vi "ShooterAngleControl.vi"(3 "error in (no error)":errorcluster, 4 "Zero":bool, 5 "Rotations":dbl) -> (0 "error out":errorcluster)   [LabVIEW 2012]
uses:
  <vilib>/Rock Robotics/WPI/CAN/Jaguar/SubVIs/WPI_CANJaguar_ControlMode.ctl
  <vilib>/Rock Robotics/WPI/CAN/Jaguar/SubVIs/WPI_CANJaguar_StatusSelect.ctl
  <vilib>/Rock Robotics/WPI/SafetyOutput/WPI_SafetyOutputConfigMenu.ctl
  <vilib>/Rock Robotics/WPI/CAN/Jaguar/SubVIs/WPI_CANJaguar_StatusChannelSelect.ctl
  Robot Global Data.vi
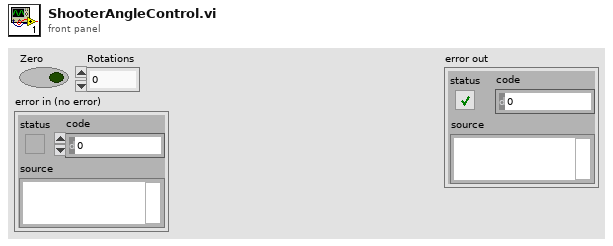
[diagram p1: front panel]
types:
  T1 = typedef "WPI_MotorControlDeviceRef.ctl" = cluster{"DeviceStatus":errorcluster, "Type":enum16{"PWM", "CAN"}, "PWM":cluster{"Digital Module":T2, "PWM Channel":T3, "DeadBand":T4}, "CAN":cluster{"Device Number":u8, "Control Mode":T5, "Semaphore":T6, "Max Vout":dbl}, "Invert":bool, "TransformRef":T7, "InvTransformRef":T7}
  T2 = typedef "FPGA_TypedefDigitalModule.ctl" = enum16{"Digital Module 1", "Digital Module 2"}
  T3 = typedef "FPGA_DIOPWMChannel.ctl" = enum8{"PWM 1", "PWM 2", "PWM 3", "PWM 4", "PWM 5", "PWM 6", "PWM 7", "PWM 8", "PWM 9", "PWM 10", "Invalid"}
  T4 = typedef "WPI_PWMDeadband.ctl" = cluster{"Name":string, "maxPositivePwm":i32, "minPositivePwm":i32, "centerPwm":i32, "maxNegativePwm":i32, "minNegativePwm":i32, "angularRange":u16}
  T5 = typedef "WPI_CANJaguar_ControlMode.ctl" = enum8{"Percent VBus", "Current", "Speed", "Position", "Voltage"}
  T6 = typedef "Semaphore RefNum" = refnum<k1>
  T7 = typedef "WPI_PWMTransform_ConPane.ctl" = refnum<vi>
  T8 = typedef "WPI_CANJaguar_StatusChannelSelect.ctl" = enum16{"Periodic Status Channel 1", "Periodic Status Channel 2", "Periodic Status Channel 3", "Periodic Status Channel 4", "On Demand Status"}
  T9 = typedef "WPI_SafetyOutputConfigMenu.ctl" = enum16{"Enable", "Disable"}
  T10 = typedef "WPI_CANJaguar_StatusSelect.ctl" = enum16{"Output Percent VBus", "Output Voltage", "Bus Voltage", "Current", "Temperature", "Position", "Speed", "Limit Switches", "Faults", "Fault Counters", "Power Cycle"}
  T11 = typedef "WPI_CANJaguar_Status.ctl" = cluster{"Output Percent VBus":dbl, "Output Voltage":dbl, "Bus Voltage":dbl, "Current":dbl, "Temperature":dbl, "Position":dbl, "Speed":dbl, "Limits":cluster{"Forward Limit":bool, "Reverse Limit":bool, "Forward Soft Limit":bool, "Reverse Soft Limit":bool, "Sticky Forward Limit":bool, "Sticky Reverse Limit":bool, "Sticky Forward Soft Limit":bool, "Sticky Reverse Soft Limit":bool}, "Faults":cluster{"Current Fault":bool, "Temperature Fault":bool, "Bus Voltage Fault":bool, "Gate Driver Fault":bool, "Comm Fault":bool}, "Fault Counters":cluster{"Current Faults":u8, "Temperature Faults":u8, "Bus Voltage Faults":u8, "Gate Driver Faults":u8, "Comm Faults":u8, "CAN Status":u8, "CAN RX Errors":u8, "CAN TX Errors":u8}, "Power Cycle":bool}
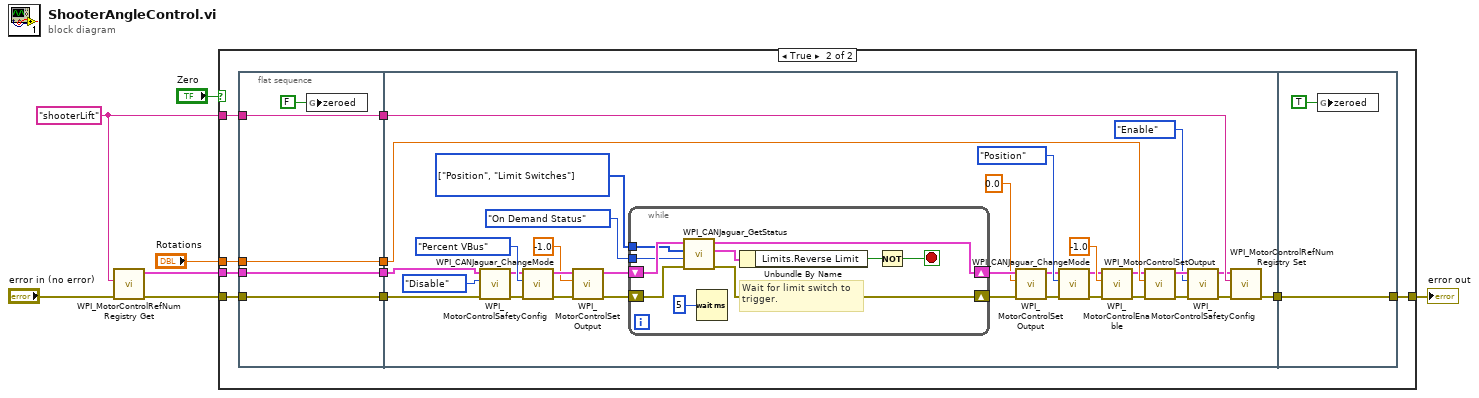
[diagram p0: block diagram]
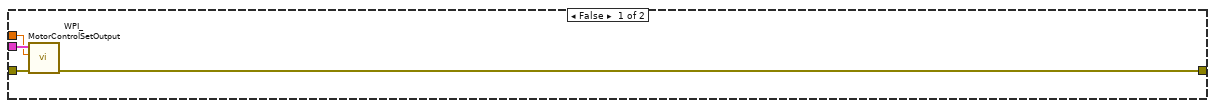
[diagram p2: hidden frame]
diagram:
  w1 = "shooterLift" ("refnum name")
  n1 = call <vilib>:"WPI_MotorControlRefNum Registry Get.vi"("error in (no error)"="error in (no error)", "refnum name"=w1) -> ("error out"=w7:errorcluster, "MotorControlDevRef"=w6:T1)  [unwired: 8 in]
  n2 = case shown="True" "Zero" {
    tunnel: w7 -> [w10 w17]
    tunnel: w6 -> [w11 w18]
    tunnel: [w9 w21] -> w3
    tunnel: "Rotations" -> [w8 w19]
    tunnel: w1 -> [_ w20]
    frame False {
      n3 = call <vilib>:"WPI_MotorControlSetOutput.vi"("error in (no error)"=w10, "Output"=w8, "MotorControlDevRef"=w11) -> ("error out"=w9:errorcluster)  [unwired: 6 in, 2 out]
    }
    frame True {
      n4 = flat-sequence {
        tunnel: w17 -> [w23]
        tunnel: w18 -> [w24]
        tunnel: w19 -> [w25]
        tunnel: w20 -> [w26]
        tunnel: [w26] -> w16
        tunnel: [w25] -> w15
        tunnel: [w24] -> w14
        tunnel: [w23] -> w13
        tunnel: w16 -> [w47]
        tunnel: w15 -> [w45]
        tunnel: w14 -> [w44]
        tunnel: w13 -> [w43]
        tunnel: [w48] -> w12
        tunnel: [w70] -> w21
        tunnel: w12 -> [w70]
        frame #0 {
          n5 = global write "Robot Global Data.vi" "zeroed"(FALSE ("zeroed")) -> ()
        }
        frame #1 {
          w52 = T10[] [enum."Position", enum."Limit Switches"] items=["Output Percent VBus", "Output Voltage", "Bus Voltage", "Current", "Temperature", "Position", "Speed", "Limit Switches", "Faults", "Fault Counters", "Power Cycle"] ("Status Select")
          n6 = call <vilib>:"WPI_MotorControlSafetyConfig.vi"("error in (no error)"=w43, "mode"=WPI_SafetyOutputConfigMenu."Disable", "MotorControlDevRef"=w44) -> ("error out"=w40:errorcluster, "MotorControlDevRef"=w41:T1)  [unwired: 7 in]
          n7 = call <vilib>:"WPI_CANJaguar_ChangeMode.vi"("error in (no error)"=w40, "Control Mode"=WPI_CANJaguar_ControlMode."Percent VBus", "CAN Jaguar Ref"=w41) -> ("error out"=w57:errorcluster, "CAN Jaguar Ref Out"=w56:T1)  [unwired: 7 in]
          n8 = call <vilib>:"WPI_MotorControlSetOutput.vi"("error in (no error)"=w57, "Output"=-1.0, "MotorControlDevRef"=w56) -> ("error out"=w54:errorcluster, "MotorControlDevRef"=w53:T1)  [unwired: 6 in, 1 out]
          n9 = while {
            tunnel: w52 -> [w65]
            shift-right: [w64] -> w49
            shift-left: w53 -> [w67]
            shift-right: [w63] -> w50
            shift-left: w54 -> [w68]
            tunnel: WPI_CANJaguar_StatusChannelSelect."On Demand Status" ("Status Channel Select") -> [w60]
            stop <- w59 stop-if-true
            # "Wait for limit switch to\ntrigger."
            n10 = call <vilib>:"WPI_CANJaguar_GetStatus.vi"("error in (no error)"=w68, "Status Channel Select"=w60, "Status Select"=w65, "CAN Jaguar Ref"=w67) -> ("error out"=w63:errorcluster, "Status"=w66:T11, "CAN Jaguar Ref Out"=w64:T1)  [unwired: 5 in]
            n11 = Wait (ms)(milliseconds to wait=u32 5) -> ()  [unwired: 1 out]
            n12 = Unbundle By Name(w66) -> ("Limits.Reverse Limit"=w61:bool)
            n13 = Not(x=w61) -> (.not. x?=w59:bool)
          }
          n14 = call <vilib>:"WPI_MotorControlSetOutput.vi"("error in (no error)"=w50, "Output"=0.0, "MotorControlDevRef"=w49) -> ("error out"=w29:errorcluster, "MotorControlDevRef"=w28:T1)  [unwired: 6 in, 1 out]
          n15 = call <vilib>:"WPI_CANJaguar_ChangeMode.vi"("error in (no error)"=w29, "Control Mode"=WPI_CANJaguar_ControlMode."Position", "CAN Jaguar Ref"=w28) -> ("error out"=w30:errorcluster, "CAN Jaguar Ref Out"=w31:T1)  [unwired: 7 in]
          n16 = call <vilib>:"WPI_MotorControlEnable.vi"("error in (no error)"=w30, "Encoder Initial Position"=-1.0, "CAN Jaguar Ref"=w31) -> ("error out"=w32:errorcluster, "CAN Jaguar Ref Out"=w33:T1)  [unwired: 7 in]
          n17 = call <vilib>:"WPI_MotorControlSetOutput.vi"("error in (no error)"=w32, "Output"=w45, "MotorControlDevRef"=w33) -> ("error out"=w38:errorcluster, "MotorControlDevRef"=w39:T1)  [unwired: 6 in, 1 out]
          n18 = call <vilib>:"WPI_MotorControlSafetyConfig.vi"("error in (no error)"=w38, "mode"=WPI_SafetyOutputConfigMenu."Enable", "MotorControlDevRef"=w39) -> ("error out"=w36:errorcluster, "MotorControlDevRef"=w37:T1)  [unwired: 7 in]
          n19 = call <vilib>:"WPI_MotorControlRefNum Registry Set.vi"("error in (no error)"=w36, "refnum name"=w47, "MotorControlDevRef"=w37) -> ("error out"=w48:errorcluster)  [unwired: 7 in, 1 out]
        }
        frame #2 {
          n20 = global write "Robot Global Data.vi" "zeroed"(TRUE ("zeroed")) -> ()
        }
      }
    }
  }
  "error out" <- w3
